vi "receiver4.vi"() -> ()   [LabVIEW 2013]
uses:
  <vilib>/sound2/lvsound2.llb/Sound Data Format.ctl
  <vilib>/sound2/lvsound2.llb/Sound File Info (path).vi
  <vilib>/sound2/lvsound2.llb/Sound File Read Open.vi
  <vilib>/sound2/lvsound2.llb/Sound File Read (DBL).vi
  <instrlib>/niUSRP/niUSRP Fetch Rx Data (CDB WDT).vi
  <vilib>/Analysis/2dsp.llb/Rational Resample (single channel, DBL).vi
  <vilib>/sound2/lvsound2.llb/Sound Output Write (DBL Single).vi
  <vilib>/express/express analysis/Spectral/Block/exnSpectralBlock spectral measurements RMS poly.vi
  <vilib>/express/express analysis/Spectral/Block/exnSpectralBlock spectral measurements RMS WFM.vi
  <vilib>/express/express analysis/Spectral/XNode/ExpressSpectralMeasurementsBlockNode.xnode
  <vilib>/Analysis/NI_AALPro.lvlib
panel:
  out "SNR":dynamicdata(graph)
  out "Instaneous SNR":dbl
  in  "number of samples 2":i32=-1
  in  "path":path
  out "output Waveform":waveform(dbl)(graph)
  out "XY Graph":cluster{dbl[], dbl[]}(graph)
  out "error out 2":errorcluster
  in  "sound format":T1={"sample rate (S/s)"=22050.0, "number of channels"=2, "bits per sample"=16}
  out "Spectrum (FFT)":cluster{"f0":dbl, "df":dbl, "magnitude":dbl[]}(graph)
  in  "stop":bool
  out "error out":errorcluster
  in  "number of samples":i64=1000
  out "coerced gain":dbl format="%#_6f"
  out "coerced carrier frequency":dbl=100000.0 format="%#_6p"
  out "coerced IQ rate":dbl=100000.0 format="%#_6p"
  in  "active antenna":string
  in  "gain":dbl format="%#_6f"
  in  "carrier frequency":dbl=100000.0 format="%#_6p"
  in  "IQ rate":dbl=100000.0 format="%#_6p"
  in  "device names":refnum<k15>
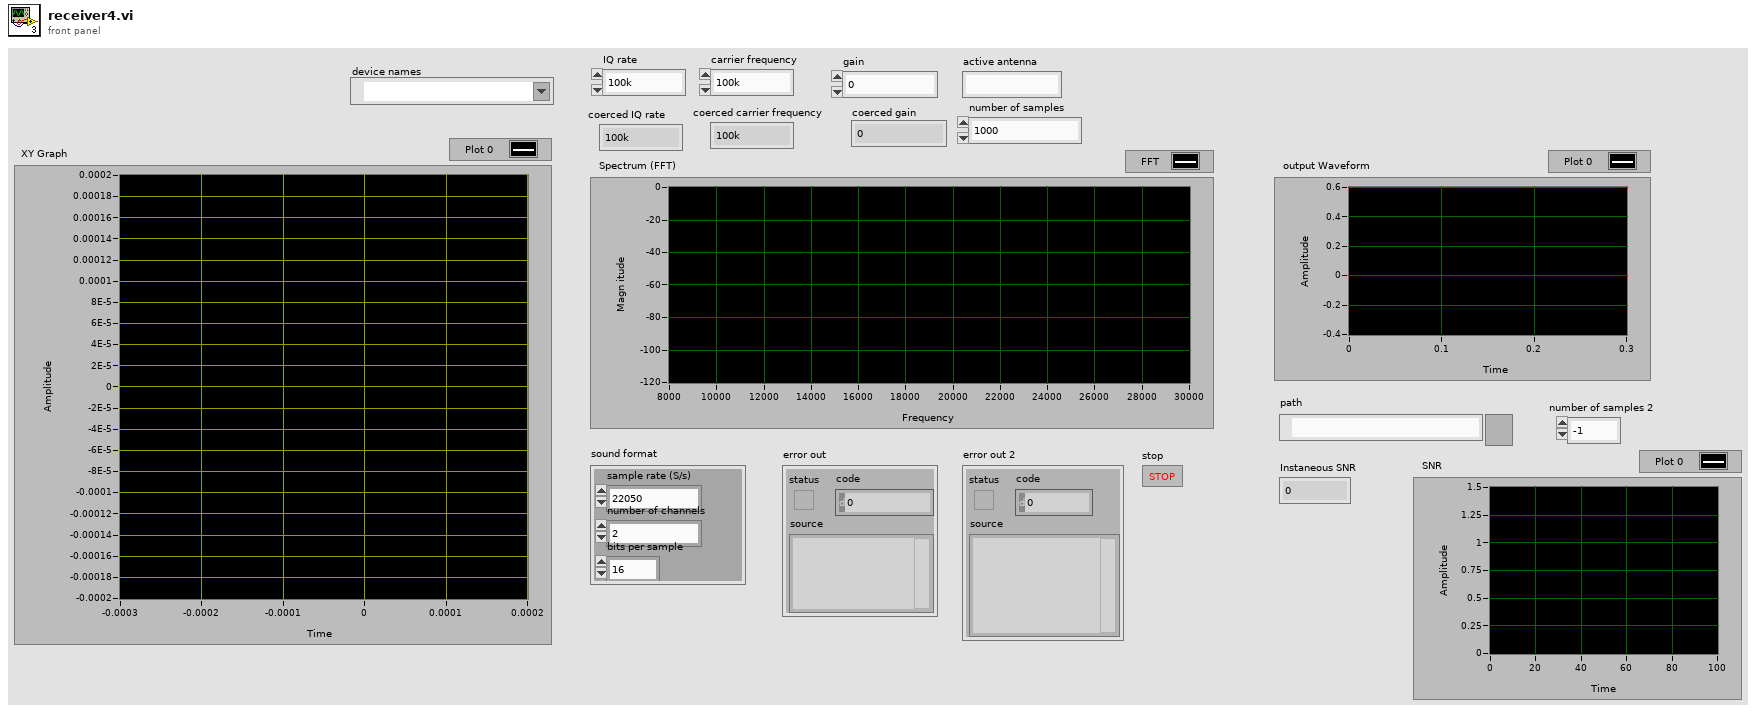
[diagram p1: front panel]
types:
  T1 = typedef "Sound Data Format.ctl" = cluster{"sample rate (S/s)":dbl, "number of channels":i32, "bits per sample":i32}
  T2 = typedef "Sound Output Task ID.ctl" = u32
  T3 = typedef "Sound File Refnum.ctl" = refnum<file>
  T4 = cluster{"averaging mode":u16, "weighting mode":u16, "number of averages":u32}
  T5 = cluster{"dB On (F)":bool, "unwrap phase (F)":bool, "convert to degree (F)":bool}
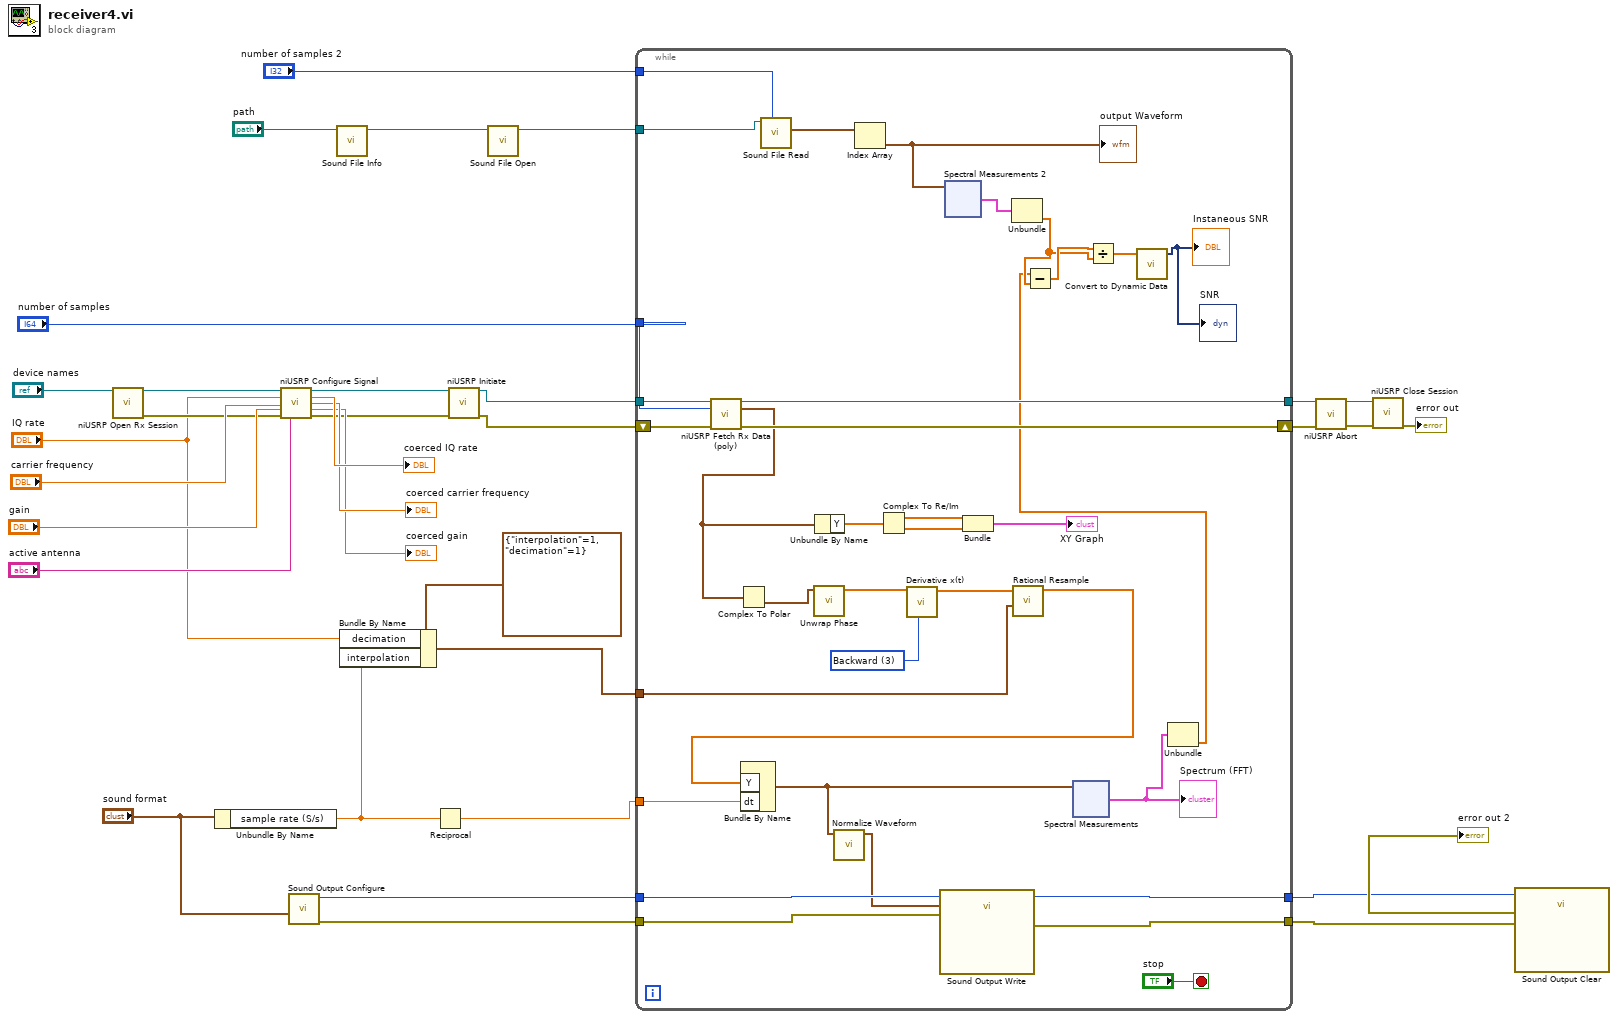
[diagram p0: block diagram]
diagram:
  n1 = call <instrlib>:"niUSRP Open Rx Session.vi"("device names"="device names") -> ("session handle out"=w16:refnum<k15>, "error out"=w17:errorcluster)  [unwired: 13 in]
  n2 = Unbundle By Name("sound format") -> ("sample rate (S/s)"=w8:dbl)
  n3 = call <instrlib>:"niUSRP Configure Signal.vi"("session handle"=w16, "IQ rate"="IQ rate", "carrier frequency"="carrier frequency", "gain"="gain", "error in (no error)"=w17, "active antenna"="active antenna") -> ("session handle out"=w28:refnum<k15>, "coerced IQ rate"=→"coerced IQ rate":dbl, "coerced carrier frequency"=→"coerced carrier frequency":dbl, "coerced gain"=→"coerced gain":dbl, "error out"=w27:errorcluster)  [unwired: 5 in]
  n4 = call <vilib>:"Sound Output Configure.vi"("sound format"="sound format") -> ("error out"=w12:errorcluster, "task ID"=w13:T2)  [unwired: 9 in]
  n5 = call-poly <vilib>:"Sound File Info.vi"("path"="path") -> ("path out"=w4:path)  [unwired: 7 in, 3 out]
  n6 = Bundle By Name(cluster=cluster{"interpolation":i32, "decimation":i32} {"interpolation"=1, "decimation"=1} ("input cluster"), "decimation"="IQ rate", "interpolation"=w8) -> (w7:cluster{"interpolation":i32, "decimation":i32})
  n7 = Reciprocal(x=w8) -> (1/x=w14:dbl)
  n8 = call <instrlib>:"niUSRP Initiate.vi"("session handle"=w28, "error in (no error)"=w27) -> ("session handle out"=w25:refnum<k15>, "error out"=w24:errorcluster)  [unwired: 12 in]
  n9 = call-poly <vilib>:"Sound File Open.vi"("path"=w4) -> ("sound file refnum"=w1:T3)  [unwired: 9 in, 1 out]
  n10 = while {
    tunnel: "number of samples" -> [w69]
    tunnel: w25 -> [w68]
    shift-right: [w65] -> w22
    shift-left: w24 -> [w67]
    tunnel: [w66] -> w23
    tunnel: w7 -> [w55]
    tunnel: w14 -> [w53]
    tunnel: w13 -> [w52]
    tunnel: w12 -> [w51]
    tunnel: [w50] -> w5
    tunnel: [w49] -> w11
    tunnel: "number of samples 2" -> [w45]
    tunnel: w1 -> [w44]
    stop <- "stop" stop-if-true
    w57 = u16 3 items=["2nd Order Central", "4th Order Central", "Forward", "Backward"] ("method")
    n11 = call-poly <instrlib>:"niUSRP Fetch Rx Data (poly).vi"("session handle"=w68, "number of samples"=w69, "error in (no error)"=w67) -> ("session handle out"=w66:refnum<k15>, "data"=w60:waveform(cdb), "error out"=w65:errorcluster)  [unwired: 9 in, 1 out]
    n12 = Complex To Polar(r * e^(i*theta)=w60) -> (theta=w59:waveform(dbl))  [unwired: 1 out]
    n13 = call-poly <vilib>:"Sound File Read.vi"("number of samples/ch (-1: all)"=w45, "sound file refnum"=w44) -> ("data"=w46:waveform(dbl)[])  [unwired: 5 in, 4 out]
    n14 = call <vilib>:"Unwrap Phase.vi"("Phase"=w59) -> ("Unwrapped Phase"=w58:dbl[])  [unwired: 9 in, 1 out]
    n15 = Unbundle By Name(w60) -> ("Y"=w63:cdb[])
    n16 = Index Array(array=w46) -> (element=w43:waveform(dbl))  [unwired: 1 in]
    "output Waveform" <- w43
    n17 = Complex To Re/Im(x + iy=w63) -> (x=w62:dbl[], y=w61:dbl[])
    n18 = call <vilib>:"Derivative x(t).vi"("method"=w57, "X"=w58) -> ("dX/dt"=w56:dbl[])  [unwired: 8 in, 1 out]
    n19 = xnode "Spectral Measurements 2"("Signals"=w43) -> ("FFT - (RMS)"=w41:cluster{"f0":dbl, "df":dbl, "magnitude":dbl[]})  [unwired: 1 in, 2 out]
    n20 = Bundle(w62, w61) -> (→"XY Graph":cluster{dbl[], dbl[]})  [unwired: 1 in]
    n21 = Unbundle(w41) -> ("magnitude"=w37:dbl[])  [unwired: 2 out]
    n22 = call-poly <vilib>:"Rational Resample.vi"("resample factor"=w55, "X"=w56) -> ("Y"=w54:dbl[])  [unwired: 7 in, 2 out]
    n23 = Bundle By Name("Y"=w54, "dt"=w53) -> (w42:waveform(dbl))  [unwired: 1 in]
    n24 = call <vilib>:"Normalize Waveform.vi"("waveform in"=w42) -> ("normalized waveform"=w47:waveform(dbl))  [unwired: 7 in, 3 out]
    n25 = call-poly <vilib>:"Sound Output Write.vi"("error in (no error)"=w51, "data"=w47, "task ID"=w52) -> ("error out"=w49:errorcluster, "task ID out"=w50:T2)  [unwired: 7 in]
    n26 = xnode "Spectral Measurements"("Signals"=w42) -> ("FFT - (RMS)"=w40:cluster{"f0":dbl, "df":dbl, "magnitude":dbl[]})  [unwired: 1 in, 2 out]
    "Spectrum (FFT)" <- w40
    n27 = Unbundle(w40) -> ("magnitude"=w36:dbl[])  [unwired: 2 out]
    n28 = Subtract(x=w36, y=w37) -> (x-y=w39:dbl[])
    n29 = Divide(x=w39, y=w37) -> (x/y=w38:dbl[])
    n30 = call "Convert to Dynamic Data"("Array"=w38) -> ("Dynamic Data Type"=→"Instaneous SNR" →"SNR":dynamicdata)  [unwired: 3 in]
  }
  n31 = call <instrlib>:"niUSRP Abort.vi"("session handle"=w23, "error in (no error)"=w22) -> ("session handle out"=w20:refnum<k15>, "error out"=w21:errorcluster)  [unwired: 12 in]
  n32 = call <instrlib>:"niUSRP Close Session.vi"("session handle"=w20, "error in (no error)"=w21) -> ("error out"=→"error out":errorcluster)  [unwired: 13 in]
  n33 = call <vilib>:"Sound Output Clear.vi"("error in (no error)"=w11, "task ID"=w5) -> ("error out"=→"error out 2":errorcluster)  [unwired: 9 in]
